vi "Cyklus.vi"() -> ()   [LabVIEW 2022 SP3]
uses:
  Coolprop_64bit/CoolProp_advanced.llb/FluidCommon.ctl
  Coolprop_64bit/CoolProp_advanced.llb/FluidOfInterest.ctl
  Coolprop_64bit/Coolprop_lib.lvlib
panel:
  out "XY Graph":cluster{dbl[], dbl[]}[](graph)
  out "point 4":T1
  out "Punkt 3":T1
  out "punkt1":T1
  out "Punkt 2":T1
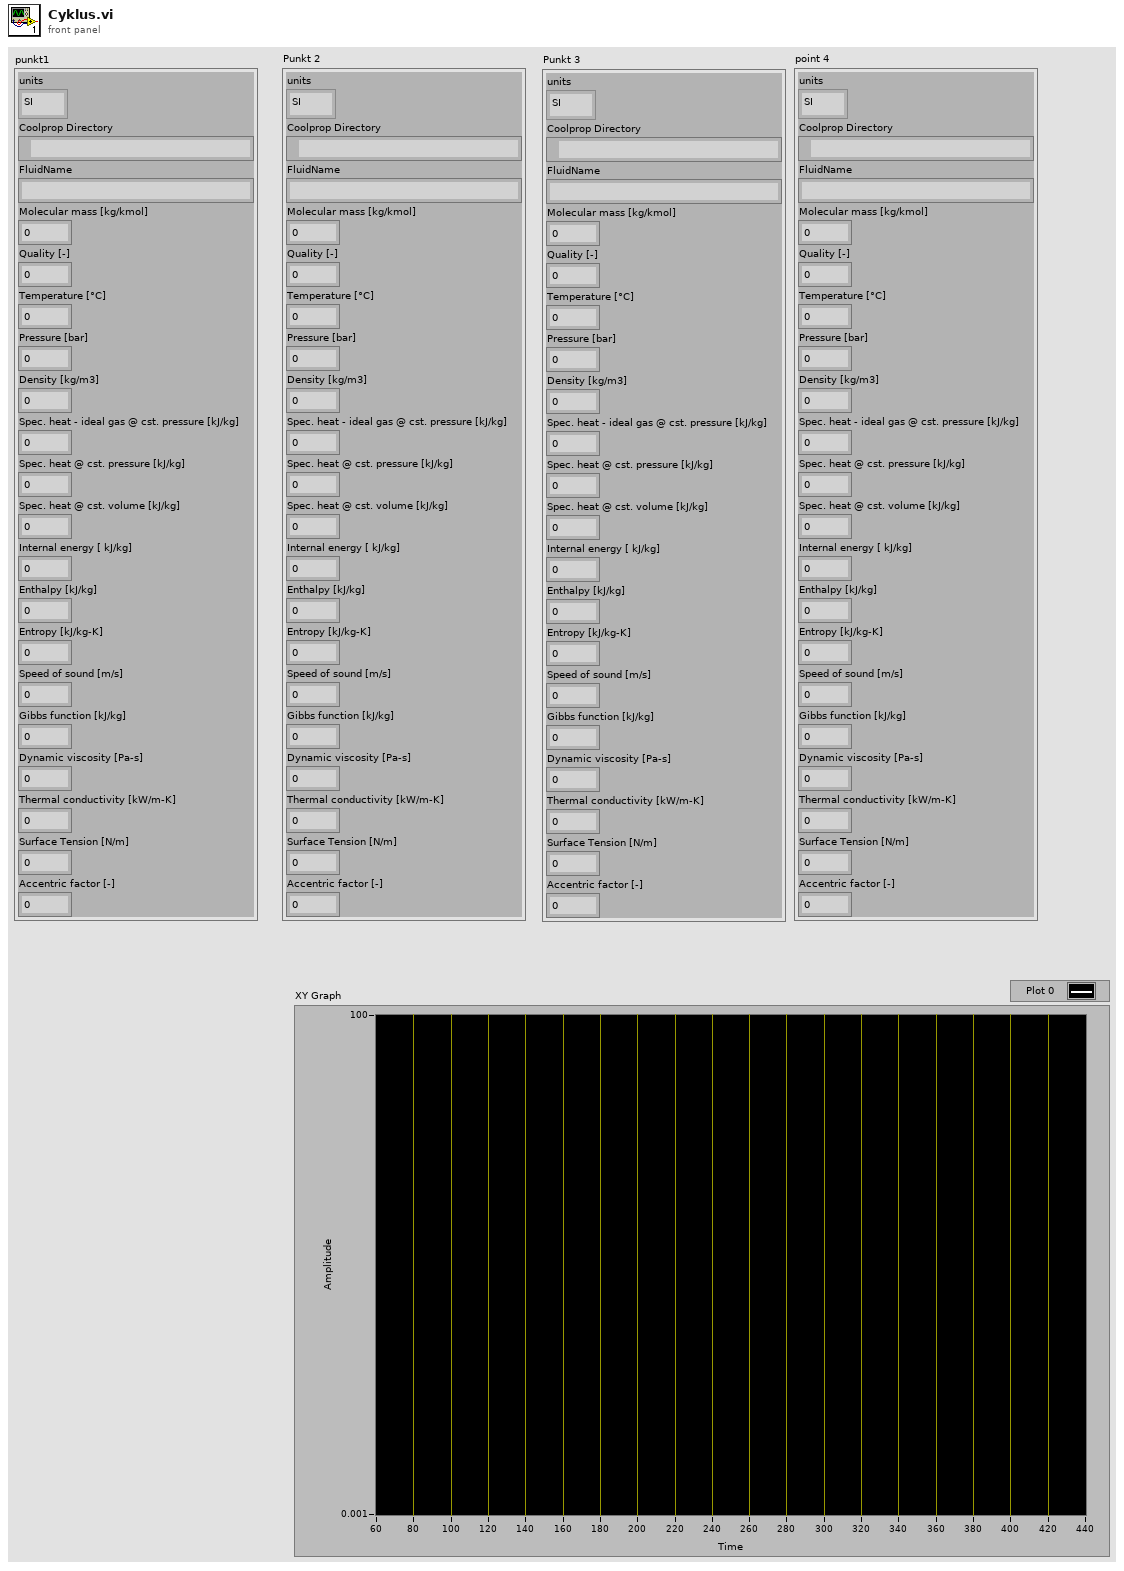
[diagram p1: front panel]
types:
  T1 = typedef "Coolprop_lib.lvlib/FluidCommon.ctl" = cluster{"units":enum16{"SI", "IP"}, "Coolprop Directory":path, "FluidName":string, "Molecular mass [kg/kmol]":dbl, "Quality [-]":dbl, "Temperature [°C]":dbl, "Pressure [bar]":dbl, "Density [kg/m3]":dbl, "Spec. heat - ideal gas @ cst. pressure [kJ/kg]":dbl, "Spec. heat @ cst. pressure [kJ/kg]":dbl, "Spec. heat @ cst. volume [kJ/kg]":dbl, "Internal energy [ kJ/kg]":dbl, "Enthalpy [kJ/kg]":dbl, "Entropy [kJ/kg-K]":dbl, "Speed of sound [m/s]":dbl, "Gibbs function [kJ/kg]":dbl, "Dynamic viscosity [Pa-s]":dbl, "Thermal conductivity [kW/m-K]":dbl, "Surface Tension [N/m]":dbl, "Accentric factor [-]":dbl}
  T2 = typedef "Coolprop_lib.lvlib/FluidOfInterest.ctl" = string
  T3 = enum16{"0", "TP", "TD", "PD", "TQ", "PQ", "HP", "SP", "SH"}
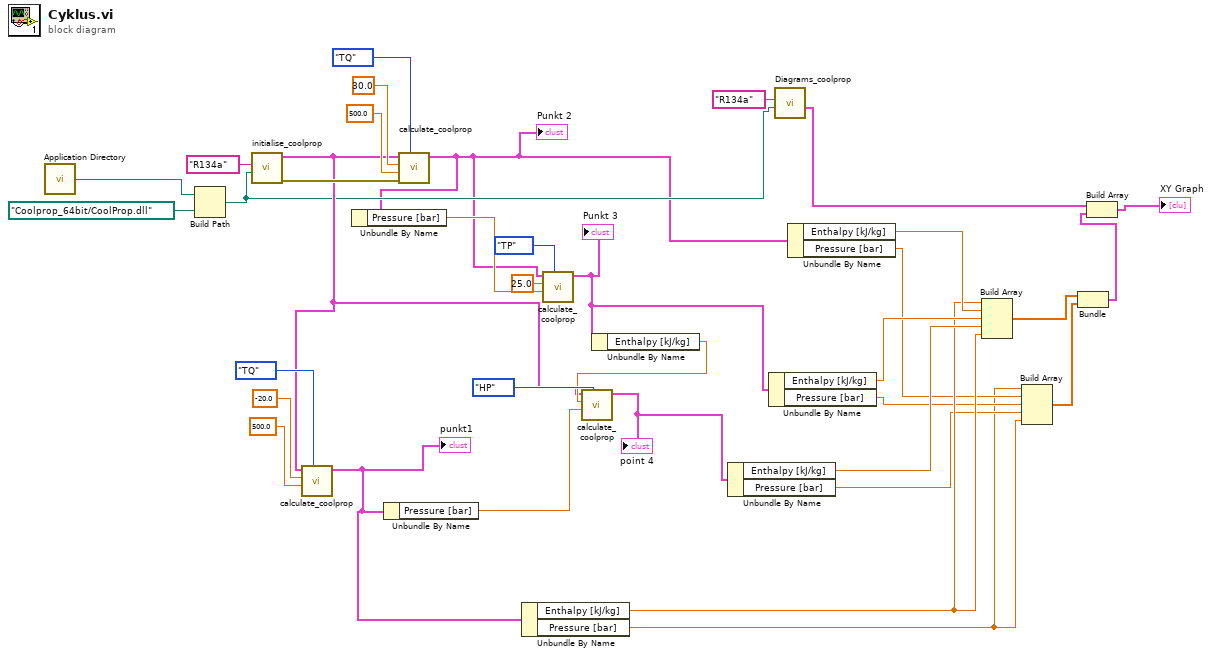
[diagram p0: block diagram]
diagram:
  n1 = call <vilib>:"Application Directory.vi"() -> ("Application Directory"=w36:path)
  n2 = Build Path(base path=w36, name or relative path=path "Coolprop_64bit/CoolProp.dll") -> (appended path=w18:path)
  n3 = call "initialise_coolprop.vi"("Path to CoolProp.dll"=w18, "FluidOfInterest"=T2 "R134a") -> ("error out"=w30:errorcluster, "Common Out"=w20:T1)  [unwired: 7 in, 1 out]
  n4 = call "calculate_coolprop.vi"("InputCode"=T3."TQ", "Input_2"=500.0, "Input_1"=-20.0, "Common In"=w20) -> ("Common Out"=w17:T1)  [unwired: 3 in, 1 out]
  "punkt1" <- w17
  n5 = Unbundle By Name(w17) -> ("Pressure [bar]"=w22:dbl)
  n6 = call "calculate_coolprop.vi"("InputCode"=T3."TQ", "error in"=w30, "Input_2"=500.0, "Input_1"=30.0, "Common In"=w20) -> ("Common Out"=w16:T1)  [unwired: 2 in, 1 out]
  "Punkt 2" <- w16
  n7 = Unbundle By Name(w16) -> ("Pressure [bar]"=w24:dbl)
  n8 = Unbundle By Name(w17) -> ("Enthalpy [kJ/kg]"=w10:dbl, "Pressure [bar]"=w6:dbl)
  n9 = call "calculate_coolprop.vi"("InputCode"=T3."TP", "Input_2"=w24, "Input_1"=25.0, "Common In"=w16) -> ("Common Out"=w15:T1)  [unwired: 3 in, 1 out]
  "Punkt 3" <- w15
  n10 = Unbundle By Name(w15) -> ("Enthalpy [kJ/kg]"=w21:dbl)
  n11 = call "calculate_coolprop.vi"("InputCode"=T3."HP", "Input_2"=w22, "Input_1"=w21, "Common In"=w20) -> ("Common Out"=w14:T1)  [unwired: 3 in, 1 out]
  "point 4" <- w14
  n12 = Unbundle By Name(w14) -> ("Enthalpy [kJ/kg]"=w11:dbl, "Pressure [bar]"=w7:dbl)
  n13 = Unbundle By Name(w15) -> ("Enthalpy [kJ/kg]"=w12:dbl, "Pressure [bar]"=w8:dbl)
  n14 = call "Diagrams_coolprop.vi"("Path"=w18, "FluidOfInterest"=T2 "R134a") -> ("ph"=w2:cluster{dbl[], dbl[]})  [unwired: 2 in, 7 out]
  n15 = Unbundle By Name(w16) -> ("Enthalpy [kJ/kg]"=w13:dbl, "Pressure [bar]"=w9:dbl)
  n16 = Build Array(w10, w13, w12, w11, w10) -> (w4:dbl[])
  n17 = Build Array(w6, w9, w8, w7, w6) -> (w5:dbl[])
  n18 = Bundle(w4, w5) -> (w3:cluster{dbl[], dbl[]})  [unwired: 1 in]
  n19 = Build Array(w2, w3) -> (→"XY Graph":cluster{dbl[], dbl[]}[])
